vi "On Close.vi"(8 "error in (no error)":errorcluster, 10 "Actor in":refnum<class "Actor.lvclass">, 11 "Client Connection Handler Msg in":refnum<class "Server Connection Handler Msg.lvclass">) -> (0 "error out":errorcluster, 2 "Actor out":refnum<class "Actor.lvclass">, 3 "Client Connection Handler Msg out":refnum<class "Server Connection Handler Msg.lvclass">)   [LabVIEW 2021, in "Echo Broadcast with External Client.lvlib" / "Server Connection Handler Msg.lvclass"]
uses:
  Server Connection Handler Msg.lvclass
  <vilib>/ActorFramework/Actor/Actor.lvclass
  WebSocket Actor/Abstract Messages/WebSocket Connection Handler Msg/WebSocket Connection Handler Msg.lvclass
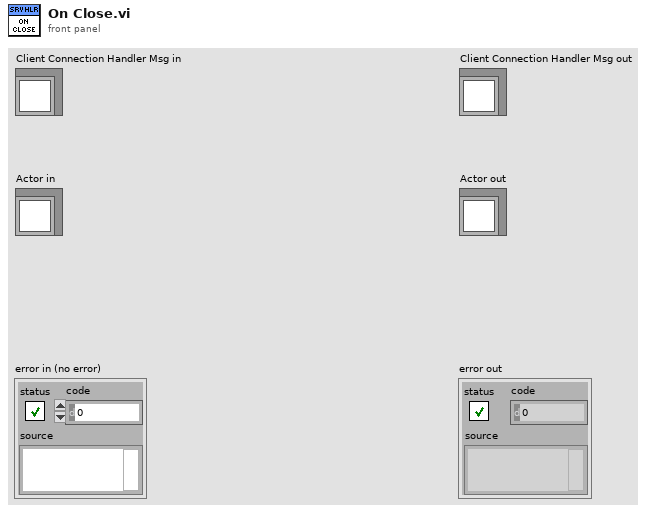
[diagram p1: front panel]
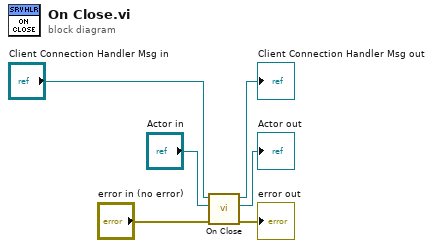
[diagram p0: block diagram]
diagram:
  n1 = call-parent "On Close.vi"("error in (no error)"="error in (no error)", "Actor in"="Actor in", "WebSocket Connection Handler Msg in"="Client Connection Handler Msg in") -> ("error out"=→"error out":errorcluster, "Actor out"=→"Actor out":refnum<class "Actor.lvclass">, "WebSocket Connection Handler Msg out"=→"Client Connection Handler Msg out":refnum<class "Server Connection Handler Msg.lvclass">)  [unwired: 6 in]
